vi "Set Visible State on Pages.vi"(8 "error in (no error)":errorcluster, 9 "Tabs Visible?":bool, 10 "Pages Visible":bool[](array[boolean]), 11 "TabControl in":refnum<vi>) -> (0 "error out":errorcluster)   [LabVIEW 2026]
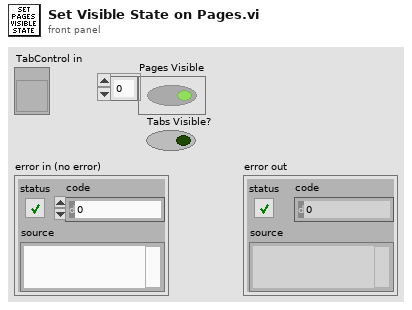
[diagram p1: front panel]
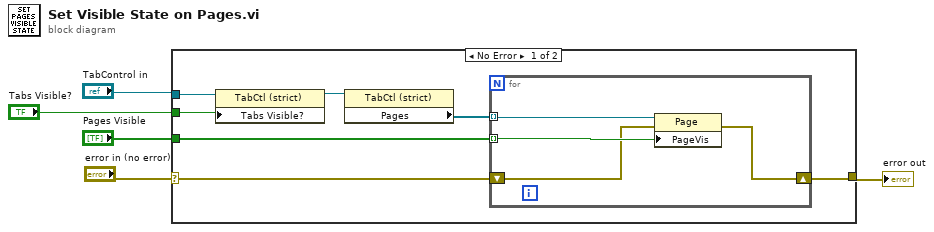
[diagram p0: block diagram]
diagram:
  n1 = case shown="No Error" "error in (no error)" {
    selector: "error in (no error)" -> [w12 w17]
    tunnel: "TabControl in" -> [w8 _]
    tunnel: [w11 w17] -> w4
    tunnel: "Pages Visible" -> [w10 _]
    tunnel: "Tabs Visible?" -> [w6 _]
    frame No Error {
      n2 = property on="Property Node" class="TabCtl (strict)"(reference=w8, "Tabs Visible?"=w6) -> (reference out=w7:refnum<vi>)  [unwired: 1 in, 1 out]
      n3 = property on="Property Node" class="TabCtl (strict)"(reference=w7) -> ("Pages"=w9:refnum<vi>[])  [unwired: 1 in, 2 out]
      n4 = for {
        shift-right: [w14] -> w11
        shift-left: w12 -> [w15]
        tunnel: w10 -> [w16] mode=indexing
        tunnel: w9 -> [w13] mode=indexing
        n5 = property class="Page"(reference=w13, error in=w15, "PageVis"=w16) -> (error out=w14:errorcluster)  [unwired: 1 out]
      }
    }
    frame Error {
    }
  }
  "error out" <- w4
